vi "Test Config Load.vi"() -> ()   [LabVIEW 2020, in "CDM-Config.lvlib"]
uses:
  CDM-Config.lvlib
  Config Manager/Config Manager.lvclass/Config Manager.ctl
  Config-JSON/Config-JSON.lvclass
  C:/dev/lv20CE/lv-cdm/CDM-Config/Config Storage/Config Storage.lvclass
  Config-INI/Config-INI.lvclass
  Config Element/Config Element.lvclass
  Config Filter/Config Lookup.lvclass
  Config Manager/Config Manager.lvclass
  Config Storage/Config Storage.lvclass
panel:
  in  "Tree":string(tree)
  out "Legio IP":string
  out "Albus IP":string
  out "error out":errorcluster
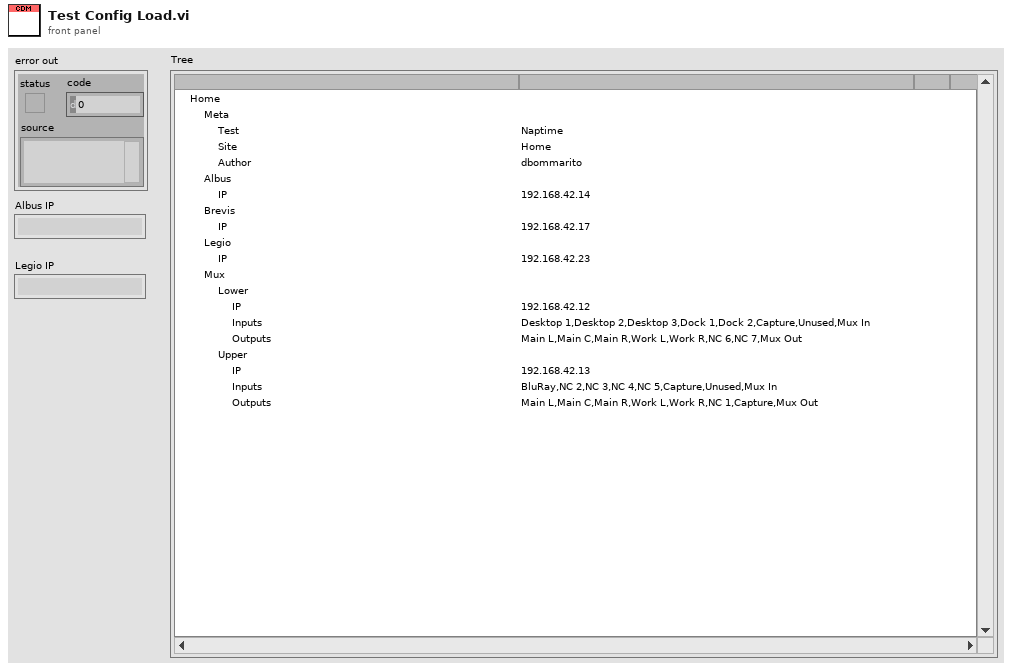
[diagram p1: front panel]
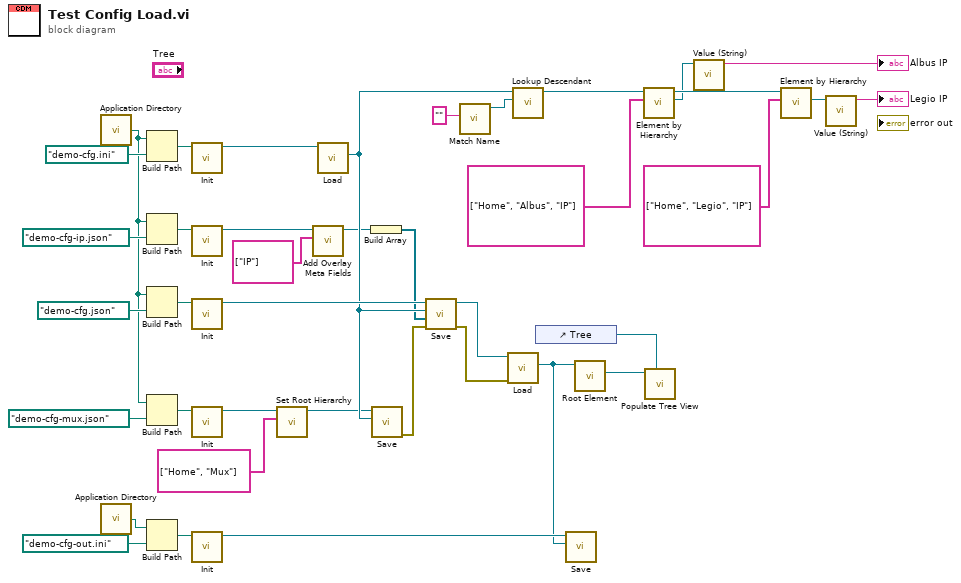
[diagram p0: block diagram]
diagram:
  n1 = call <vilib>:"Application Directory.vi"() -> ("Application Directory"=w12:path)
  n2 = call <vilib>:"Application Directory.vi"() -> ("Application Directory"=w28:path)
  n3 = Build Path(base path=w12, name or relative path=path "demo-cfg.ini") -> (appended path=w37:path)
  n4 = Build Path(base path=w12, name or relative path=path "demo-cfg-ip.json") -> (appended path=w14:path)
  n5 = Build Path(base path=w12, name or relative path=path "demo-cfg.json") -> (appended path=w29:path)
  n6 = Build Path(base path=w12, name or relative path=path "demo-cfg-mux.json") -> (appended path=w16:path)
  n7 = Build Path(base path=w28, name or relative path=path "demo-cfg-out.ini") -> (appended path=w27:path)
  n8 = call "Init.vi"("INI Path"=w37) -> ("Config-INI out"=w21:refnum<class "Config-INI.lvclass">)  [unwired: 9 in, 1 out]
  n9 = call "Init.vi"("Path"=w14) -> ("Config-JSON out"=w11:refnum<class "Config-JSON.lvclass">)  [unwired: 9 in, 1 out]
  n10 = call "Init.vi"("Path"=w29) -> ("Config-JSON out"=w19:refnum<class "Config-JSON.lvclass">)  [unwired: 9 in, 1 out]
  n11 = call "Init.vi"("Path"=w16) -> ("Config-JSON out"=w15:refnum<class "Config-JSON.lvclass">)  [unwired: 9 in, 1 out]
  n12 = call "Init.vi"("INI Path"=w27) -> ("Config-INI out"=w20:refnum<class "Config-INI.lvclass">)  [unwired: 9 in, 1 out]
  n13 = call "Set Root Hierarchy.vi"("Root Hierarchy"=string[] ["Home", "Mux"] ("Subtree Root (Entire Tree)"), "Config Storage in"=w15) -> ("Config Storage out"=w7:refnum<class "Config-JSON.lvclass">)  [unwired: 8 in, 1 out]
  n14 = call "Add Overlay Meta Fields.vi"("Meta Fields"=string[] ["IP"], "Config Storage in"=w11) -> ("Config Storage out"=w9:refnum<class "Config-JSON.lvclass">)  [unwired: 8 in, 1 out]
  n15 = call "Load.vi"("Config Storage in"=w21) -> ("Config"=w18:refnum<class "Config Manager.lvclass">)  [unwired: 8 in, 2 out]
  n16 = Build Array(w9) -> (w8:refnum<class "Config-JSON.lvclass">[])
  n17 = call "Save.vi"("Config"=w18, "Config Storage in"=w7) -> ("error out"=w2:errorcluster)  [unwired: 8 in, 1 out]
  n18 = call "Save.vi"("error in (no error)"=w2, "Overlays (None)"=w8, "Config"=w18, "Config Storage in"=w19) -> ("error out"=w39:errorcluster, "Config Storage out"=w5:refnum<class "Config-JSON.lvclass">)  [unwired: 6 in]
  n19 = call "Match Name.vi"("Name"="") -> ("Config Lookup out"=w35:refnum<class "Config Lookup.lvclass">)  [unwired: 9 in, 1 out]
  n20 = call "Load.vi"("error in (no error)"=w39, "Config Storage in"=w5) -> ("Config"=w1:refnum<class "Config Manager.lvclass">)  [unwired: 7 in, 2 out]
  n21 = call "Lookup Descendant.vi"("Lookup"=w35, "Config Manager in"=w18) -> ("Config Manager out"=w25:refnum<class "Config Manager.lvclass">)  [unwired: 7 in, 2 out]
  n22 = control-ref of="Tree"() -> (w3:refnum<vi>)
  n23 = call "Save.vi"("Config"=w1, "Config Storage in"=w20) -> ()  [unwired: 8 in, 2 out]
  n24 = call "Root Element.vi"("Config Manager in"=w1) -> ("Root Element"=w4:refnum<class "Config Element.lvclass">)  [unwired: 8 in, 2 out]
  n25 = call "Element by Hierarchy.vi"("Hierarchy"=string[] ["Home", "Albus", "IP"], "Config Manager in"=w25) -> ("Config Element"=w22:refnum<class "Config Element.lvclass">, "Config Manager out"=w24:refnum<class "Config Manager.lvclass">)  [unwired: 7 in, 1 out]
  n26 = call "Populate Tree View.vi"("Tree"=w3, "Element"=w4) -> ()  [unwired: 9 in, 1 out]
  n27 = call "Value (String).vi"("Config Element in"=w22) -> ("String Value"=→"Albus IP":string)  [unwired: 9 in, 1 out]
  n28 = call "Element by Hierarchy.vi"("Hierarchy"=string[] ["Home", "Legio", "IP"], "Config Manager in"=w24) -> ("Config Element"=w32:refnum<class "Config Element.lvclass">)  [unwired: 7 in, 2 out]
  n29 = call "Value (String).vi"("Config Element in"=w32) -> ("String Value"=→"Legio IP":string)  [unwired: 9 in, 1 out]
